vi "CRYCalc Wave & Wave Unit.vi"(8 "Work in":u16(slide), 9 "Operator":u16(ring) items=["+", "--", "x", "/"], 10 "Wave in_2":T1={"Waveform"={"X0"=0.0, "dX"=0.0, "Y"=[]}, "X data"=1, "Y data"=1, "Y axis"=1, "X unit"="s", "Y unit"="V", "Y dB ref"=1.0, "display Y"=TRUE, "display X"=TRUE, "Overload?"=FALSE, "Test Info"="", "Step No."=0, "Name"="", "protected"=FALSE, "Sqc history"=[], "Signal Channel ID"=0, "Plot Settings"={"Color"=0, "Interpolation"=0, "Point Style"=0, "Line Style"=0, "Point Color"=0, "Line Width"=0, "Bar Plot Style"=0, "Fill To"=0}, "AutoProtect"=FALSE} {"Y dB ref" format="%.1f"; "Y axis" items=["Log", "Lin"]; "Y data" items=["dB", "Lin"]; "X data" items=["dB", "Lin"]}, 11 "Wave in_1":T1={"Waveform"={"X0"=0.0, "dX"=0.0, "Y"=[]}, "X data"=1, "Y data"=1, "Y axis"=1, "X unit"="s", "Y unit"="V", "Y dB ref"=1.0, "display Y"=TRUE, "display X"=TRUE, "Overload?"=FALSE, "Test Info"="", "Step No."=0, "Name"="", "protected"=FALSE, "Sqc history"=[], "Signal Channel ID"=0, "Plot Settings"={"Color"=0, "Interpolation"=0, "Point Style"=0, "Line Style"=0, "Point Color"=0, "Line Width"=0, "Bar Plot Style"=0, "Fill To"=0}, "AutoProtect"=FALSE} {"Y dB ref" format="%.1f"; "Y axis" items=["Log", "Lin"]; "Y data" items=["dB", "Lin"]; "X data" items=["dB", "Lin"]}) -> (0 "Y data":u16, 1 "Y dB ref":dbl, 2 "X unit":string, 3 "Y unit":string)   [LabVIEW 2013]
uses:
  Typedef Control/CRYWaveform Cluster.ctl
  CRYPost Processing Global.vi
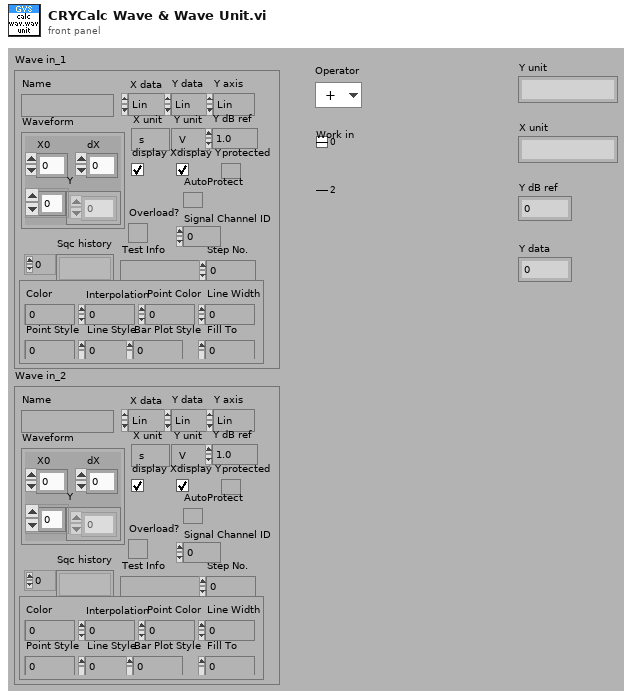
[diagram p1: front panel]
types:
  T1 = typedef "CRYWaveform Cluster.ctl" = cluster{"Waveform":cluster{"X0":dbl, "dX":dbl, "Y":sgl[]}, "X data":u16, "Y data":u16, "Y axis":u16, "X unit":string, "Y unit":string, "Y dB ref":dbl, "display Y":bool, "display X":bool, "Overload?":bool, "Test Info":string, "Step No.":i32, "Name":string, "protected":bool, "Sqc history":string[], "Signal Channel ID":i32, "Plot Settings":cluster{"Color":u32, "Interpolation":u8, "Point Style":u8, "Line Style":u8, "Point Color":u32, "Line Width":u8, "Bar Plot Style":u8, "Fill To":i16}, "AutoProtect":bool}
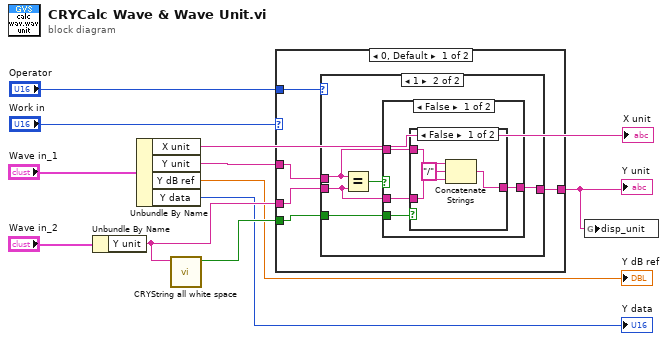
[diagram p0: block diagram]
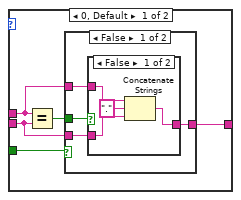
[diagram p2: hidden frame]
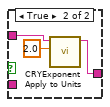
[diagram p3: hidden frame]
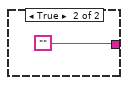
[diagram p6: hidden frame]
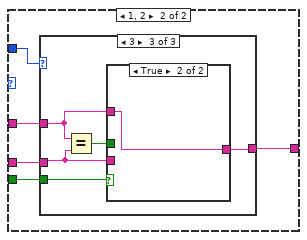
[diagram p7: hidden frame]
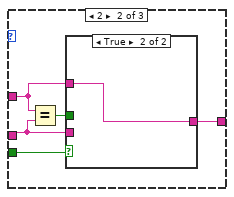
[diagram p9: hidden frame]
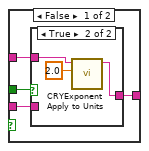
[diagram p10: hidden frame]
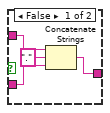
[diagram p11: hidden frame]
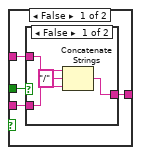
[diagram p12: hidden frame]
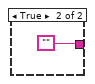
[diagram p13: hidden frame]
diagram:
  n1 = Unbundle By Name("Wave in_2") -> ("Y unit"=w6:string)
  n2 = Unbundle By Name("Wave in_1") -> ("X unit"=→"X unit":string, "Y unit"=w7:string, "Y dB ref"=→"Y dB ref":dbl, "Y data"=→"Y data":u16)
  n3 = call "CRYString all white space.vi"("String"=w6) -> ("Nothing but white space?"=w5:bool)  [unwired: 10 in]
  n4 = case shown="0, Default" "Work in" {
    tunnel: "Operator" -> [w16 w53]
    tunnel: w7 -> [w15 w52]
    tunnel: w6 -> [w13 w51]
    tunnel: [w14 w50] -> w1
    tunnel: w5 -> [w12 w49]
    frame 0, Default {
      n5 = case shown="1" w16 {
        tunnel: w15 -> [w20 w37]
        tunnel: w13 -> [w18 w36]
        tunnel: [w19 w35] -> w14
        tunnel: w12 -> [w17 w34]
        frame 0, Default {
          n6 = Equal?(x=w20, y=w18) -> (x = y?=w21:bool)
          n7 = case shown="False" w17 {
            tunnel: w21 -> [w25 _]
            tunnel: w20 -> [w24 w33]
            tunnel: [w23 w33] -> w19
            tunnel: w18 -> [w22 _]
            frame False {
              n8 = case shown="False" w25 {
                tunnel: w24 -> [w29 w31]
                tunnel: [w26 w30] -> w23
                tunnel: w22 -> [w28 _]
                frame False {
                  n9 = Concatenate Strings(w29, "." ("string"), w28) -> (w26:string)
                }
                frame True {
                  n10 = call "CRYExponent Apply to Units.vi"("Exponent to apply"=2.0, "Unit in"=w31) -> ("Unit out"=w30:string)  [unwired: 9 out]
                }
              }
            }
            frame True {
            }
          }
        }
        frame 1 {
          n11 = Equal?(x=w37, y=w36) -> (x = y?=w38:bool)
          n12 = case shown="False" w38 {
            tunnel: w37 -> [w42 _]
            tunnel: [w40 ""] -> w35
            tunnel: w36 -> [w41 _]
            tunnel: w34 -> [w39 _]
            frame False {
              n13 = case shown="False" w39 {
                tunnel: w42 -> [w46 w47]
                tunnel: w41 -> [w45 _]
                tunnel: [w43 w47] -> w40
                frame False {
                  n14 = Concatenate Strings(w46, "/" ("string"), w45) -> (w43:string)
                }
                frame True {
                }
              }
            }
            frame True {
            }
          }
        }
      }
    }
    frame 1, 2 {
      n15 = case shown="3" w53 {
        tunnel: w52 -> [w54 w58 w75]
        tunnel: w51 -> [_ w57 w74]
        tunnel: [w54 w56 w73] -> w50
        tunnel: w49 -> [_ w55 w72]
        frame 0, 1, Default {
        }
        frame 2 {
          n16 = Equal?(x=w58, y=w57) -> (x = y?=w59:bool)
          n17 = case shown="True" w55 {
            tunnel: w59 -> [w63 _]
            tunnel: w58 -> [w62 w71]
            tunnel: w57 -> [w61 _]
            tunnel: [w60 w71] -> w56
            frame False {
              n18 = case shown="True" w63 {
                tunnel: w62 -> [w67 w69]
                tunnel: [w64 w68] -> w60
                tunnel: w61 -> [w66 _]
                frame False {
                  n19 = Concatenate Strings(w67, "." ("string"), w66) -> (w64:string)
                }
                frame True {
                  n20 = call "CRYExponent Apply to Units.vi"("Exponent to apply"=2.0, "Unit in"=w69) -> ("Unit out"=w68:string)  [unwired: 9 out]
                }
              }
            }
            frame True {
            }
          }
        }
        frame 3 {
          n21 = Equal?(x=w75, y=w74) -> (x = y?=w76:bool)
          n22 = case shown="True" w72 {
            tunnel: w76 -> [w80 _]
            tunnel: w75 -> [w79 w86]
            tunnel: w74 -> [w78 _]
            tunnel: [w77 w86] -> w73
            frame False {
              n23 = case shown="False" w80 {
                tunnel: w79 -> [w84 _]
                tunnel: [w81 ""] -> w77
                tunnel: w78 -> [w83 _]
                frame False {
                  n24 = Concatenate Strings(w84, "/" ("string"), w83) -> (w81:string)
                }
                frame True {
                }
              }
            }
            frame True {
            }
          }
        }
      }
    }
  }
  "Y unit" <- w1
  n25 = global write "CRYPost Processing Global.vi" "disp_unit"(w1) -> ()
